vi "negate-threshold 1.vi"() -> ()   [LabVIEW 2009]
uses:
  <vilib>/vision/NI_Vision_Development_Module.lvlib
panel:
  in  "stop":bool=TRUE
  in  "load1 Button":bool
  in  "Negate  Button":bool
  in  "Save Button":bool
  in  "Threshold Button":bool
  in  "Threshold Values":T1(slide)={"Minimum Value"=0.0, "Maximum Value"=99.65958} scale=0.0..255.0
  in  "Keep/Replace Value (Replace)":bool=TRUE
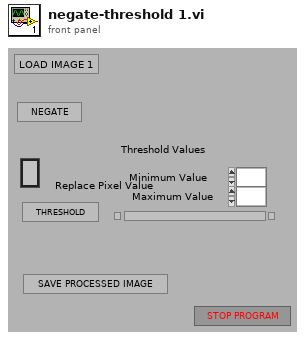
[diagram p1: front panel]
types:
  T1 = cluster{"Minimum Value":sgl, "Maximum Value":sgl}
  T2 = typedef "IMAQ Image.ctl" = refnum<image>
  T3 = enum32{"existing file", "new file", "new or existing file", "existing dir", "new dir", "new or existing dir", "existing file (use LLBs)", "new file (use LLBs)", "new or existing file (use LLBs)", "new or existing file or directory (use LLBs)", "existing dir (use LLBs)", "new dir (use LLBs)", "new or existing dir (use LLBs)", "existing file or dir", "new file or dir", "new or existing file or dir", "existing file or dir (use LLBs)", "new file or dir (use LLBs)"}
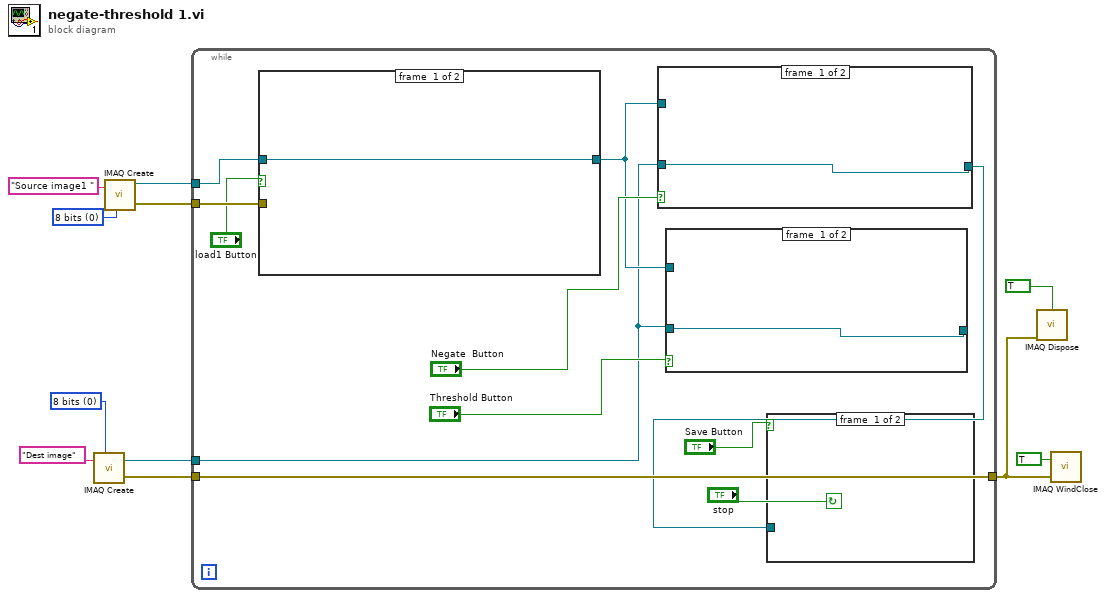
[diagram p0: block diagram]
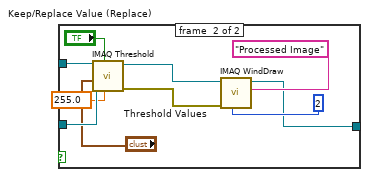
[diagram p2: hidden frame]
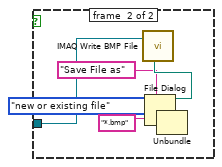
[diagram p3: hidden frame]
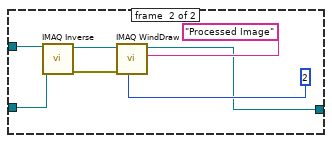
[diagram p4: hidden frame]
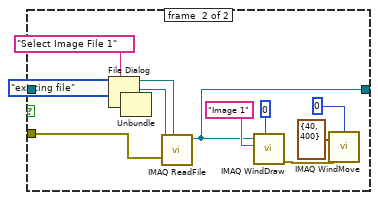
[diagram p5: hidden frame]
diagram:
  w6 = u32 0 items=["8 bits", "16 bits", "Float", "Complex", "RGB", "HSL"] ("Image Type")
  w8 = u32 0 items=["8 bits", "16 bits", "Float", "Complex", "RGB", "HSL"] ("Image Type")
  n1 = call "IMAQ Create"("Image Name"="Dest image", "Image Type"=w6) -> ("New Image"=w1:T2, "error out"=w5:errorcluster)  [unwired: 3 in]
  n2 = call "IMAQ Create"("Image Name"="Source image1 ", "Image Type"=w8) -> ("New Image"=w10:T2, "error out"=w11:errorcluster)  [unwired: 3 in]
  n3 = while {
    tunnel: w11 -> [w20]
    tunnel: w10 -> [w22]
    tunnel: w5 -> [w17]
    tunnel: [w17] -> w4
    tunnel: w1 -> [w12]
    stop <- "stop" continue-if-true
    n4 = case shown="真" "load1 Button" {
      tunnel: w22 -> [w47 w50]
      tunnel: [w47 w49] -> w13
      tunnel: w20 -> [_ w51]
      frame #0 {
      }
      frame #1 {
        (unwired) T3."existing file" ("select mode (2)")
        n5 = File Dialog(7:"Select Image File 1" ("prompt")) -> (0:w48:errorcluster, 3:w58:path)  [unwired: 6 in, 2 out]
        n6 = Unbundle(w48) -> ()  [unwired: 3 out]
        n7 = call "IMAQ ReadFile"("File Path"=w58, "error in (no error)"=w51, "Image"=w50) -> ("Image Out"=w49:T2)  [unwired: 4 in, 4 out]
        n8 = call "IMAQ WindDraw"("Window Number (0...15)"=0, "Title"="Image 1", "Image"=w49) -> ("error out"=w54:errorcluster)  [unwired: 7 in, 1 out]
        n9 = call "IMAQ WindMove"("Window Number (0...15)"=0, "Coordinates (screen)"=cluster{"X Position":i32, "Y Position":i32} {"X Position"=40, "Y Position"=400}, "error in (no error)"=w54) -> ()  [unwired: 2 in, 2 out]
      }
    }
    n10 = case shown="真" "Negate  Button" {
      tunnel: w12 -> [w39 w42]
      tunnel: [w39 w44] -> w15
      tunnel: w13 -> [_ w43]
      frame #0 {
      }
      frame #1 {
        n11 = call "IMAQ Inverse"("Image Dst"=w42, "Image Src"=w43) -> ("error out"=w40:errorcluster, "Image Dst Out"=w41:T2)  [unwired: 8 in]
        n12 = call "IMAQ WindDraw"("Window Number (0...15)"=2, "error in (no error)"=w40, "Title"="Processed Image", "Image"=w41) -> ("Image Out (duplicate)"=w44:T2)  [unwired: 6 in, 1 out]
      }
    }
    n13 = case shown="真" "Threshold Button" {
      tunnel: w12 -> [w23 w29]
      tunnel: [w23 w31] -> _
      tunnel: w13 -> [_ w30]
      frame #0 {
      }
      frame #1 {
        n14 = call "IMAQ Threshold"("Replace Value"=sgl 255.0, "Keep/Replace Value (Replace)"="Keep/Replace Value (Replace)", "Range"="Threshold Values", "Image Dst"=w29, "Image Src"=w30) -> ("error out"=w27:errorcluster, "Image Dst Out"=w28:T2)  [unwired: 5 in]
        n15 = call "IMAQ WindDraw"("Window Number (0...15)"=2, "error in (no error)"=w27, "Title"="Processed Image", "Image"=w28) -> ("Image Out (duplicate)"=w31:T2)  [unwired: 6 in, 1 out]
      }
    }
    n16 = case shown="真" "Save Button" {
      tunnel: w15 -> [_ w35]
      frame #0 {
      }
      frame #1 {
        (unwired) T3."new or existing file" ("select mode (2)")
        n17 = File Dialog(6:"*.bmp" ("pattern"), 7:"Save File as" ("prompt")) -> (0:w34:errorcluster, 3:w38:path)  [unwired: 5 in, 2 out]
        n18 = call "IMAQ Write BMP File"("File Path"=w38, "Image"=w35) -> ()  [unwired: 6 in, 1 out]
        n19 = Unbundle(w34) -> ()  [unwired: 3 out]
      }
    }
  }
  n20 = call "IMAQ Dispose"("All Images? (No)"=TRUE, "error in (no error)"=w4) -> ()  [unwired: 4 in, 1 out]
  n21 = call "IMAQ WindClose"("Close All Windows (False)"=TRUE, "error in (no error)"=w4) -> ()  [unwired: 4 in, 1 out]
